vi "PotRounding.vi"(1 "Potentiometer":dbl, 2 "Invert?":bool) -> (0 "shooter output":dbl)   [LabVIEW 2012]
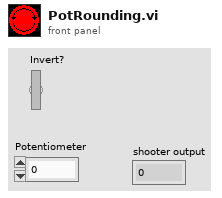
[diagram p1: front panel]
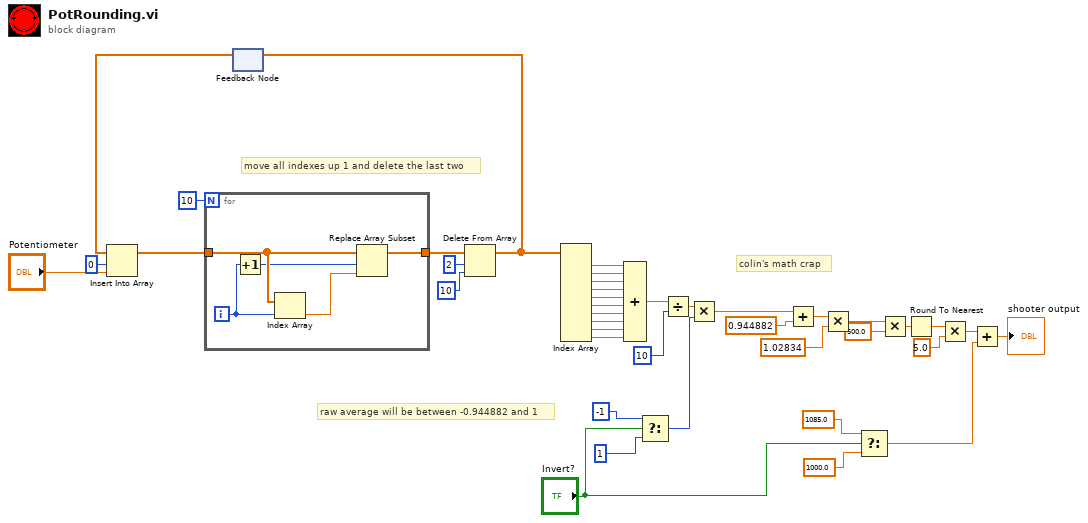
[diagram p0: block diagram]
diagram:
  # "move all indexes up 1 and delete the last two"
  # "colin's math crap"
  # "raw average will be between -0.944882 and 1"
  n1 = feedback #1() -> (w11:dbl[])  [unwired: 1 in]
  n2 = Insert Into Array(array=w11, index=0, new element="Potentiometer") -> (w39:dbl[])
  n3 = for {
    N: 10 -> [_]
    tunnel: w39 -> [w44]
    tunnel: [w41] -> w38
    i -> [w45]
    n4 = Increment(x=w45) -> (x+1=w43:i32)
    n5 = Index Array(array=w44, index=w45) -> (element=w42:dbl)
    n6 = Replace Array Subset(array=w44, new element=w42, index=w43) -> (w41:dbl[])
  }
  n7 = Delete From Array(array=w38, length=2, index=10) -> (array with subset deleted=w10:dbl[])  [unwired: 1 out]
  n8 = feedback-in #1(w10) -> ()
  n9 = Index Array(array=w10) -> (element #1=w26:dbl, element #2=w27:dbl, element #3=w28:dbl, element #4=w29:dbl, element #5=w30:dbl, element #6=w31:dbl, element #7=w32:dbl, element #8=w33:dbl, element #9=w34:dbl, element #10=w35:dbl)  [unwired: 10 in]
  n10 = Compound Arithmetic op=ADD(w26, w27, w28, w29, w30, w31, w32, w33, w34, w35) -> (w25:dbl)
  n11 = Select(t=-1, s="Invert?", f=1) -> (s? t:f=w5:i32)
  n12 = Divide(x=w25, y=10) -> (x/y=w9:dbl)
  n13 = Multiply(x=w9, y=w5) -> (x*y=w8:dbl)
  n14 = Add(x=w8, y=0.944882) -> (x+y=w15:dbl)
  n15 = Multiply(x=w15, y=1.02834 ("x")) -> (x*y=w16:dbl)
  n16 = Select(t=1085.0 ("y"), s="Invert?", f=1000.0) -> (s? t:f=w1:dbl)
  n17 = Multiply(x=w16, y=500.0) -> (x*y=w21:dbl)
  n18 = Round To Nearest(number=w21) -> (nearest integer value=w20:dbl)
  n19 = Multiply(x=w20, y=5.0) -> (x*y=w18:dbl)
  n20 = Add(x=w18, y=w1) -> (x+y=→"shooter output":dbl)
